vi "Plot strain.vi"() -> ()   [LabVIEW 2015]
uses:
  <vilib>/Utility/file.llb/Read Delimited Spreadsheet (DBL).vi
panel:
  in  "Tab Control":enum32{"Individua strain", "Total strain"}(tab)
  out "XY Graph":cluster{dbl[], "all rows":dbl[]}[](graph)
  out "XY Graph 2":cluster{dbl[], "all rows":dbl[]}[](graph)
  in  "Strain bolt number":i32
  in  "Array":path[](array[path])
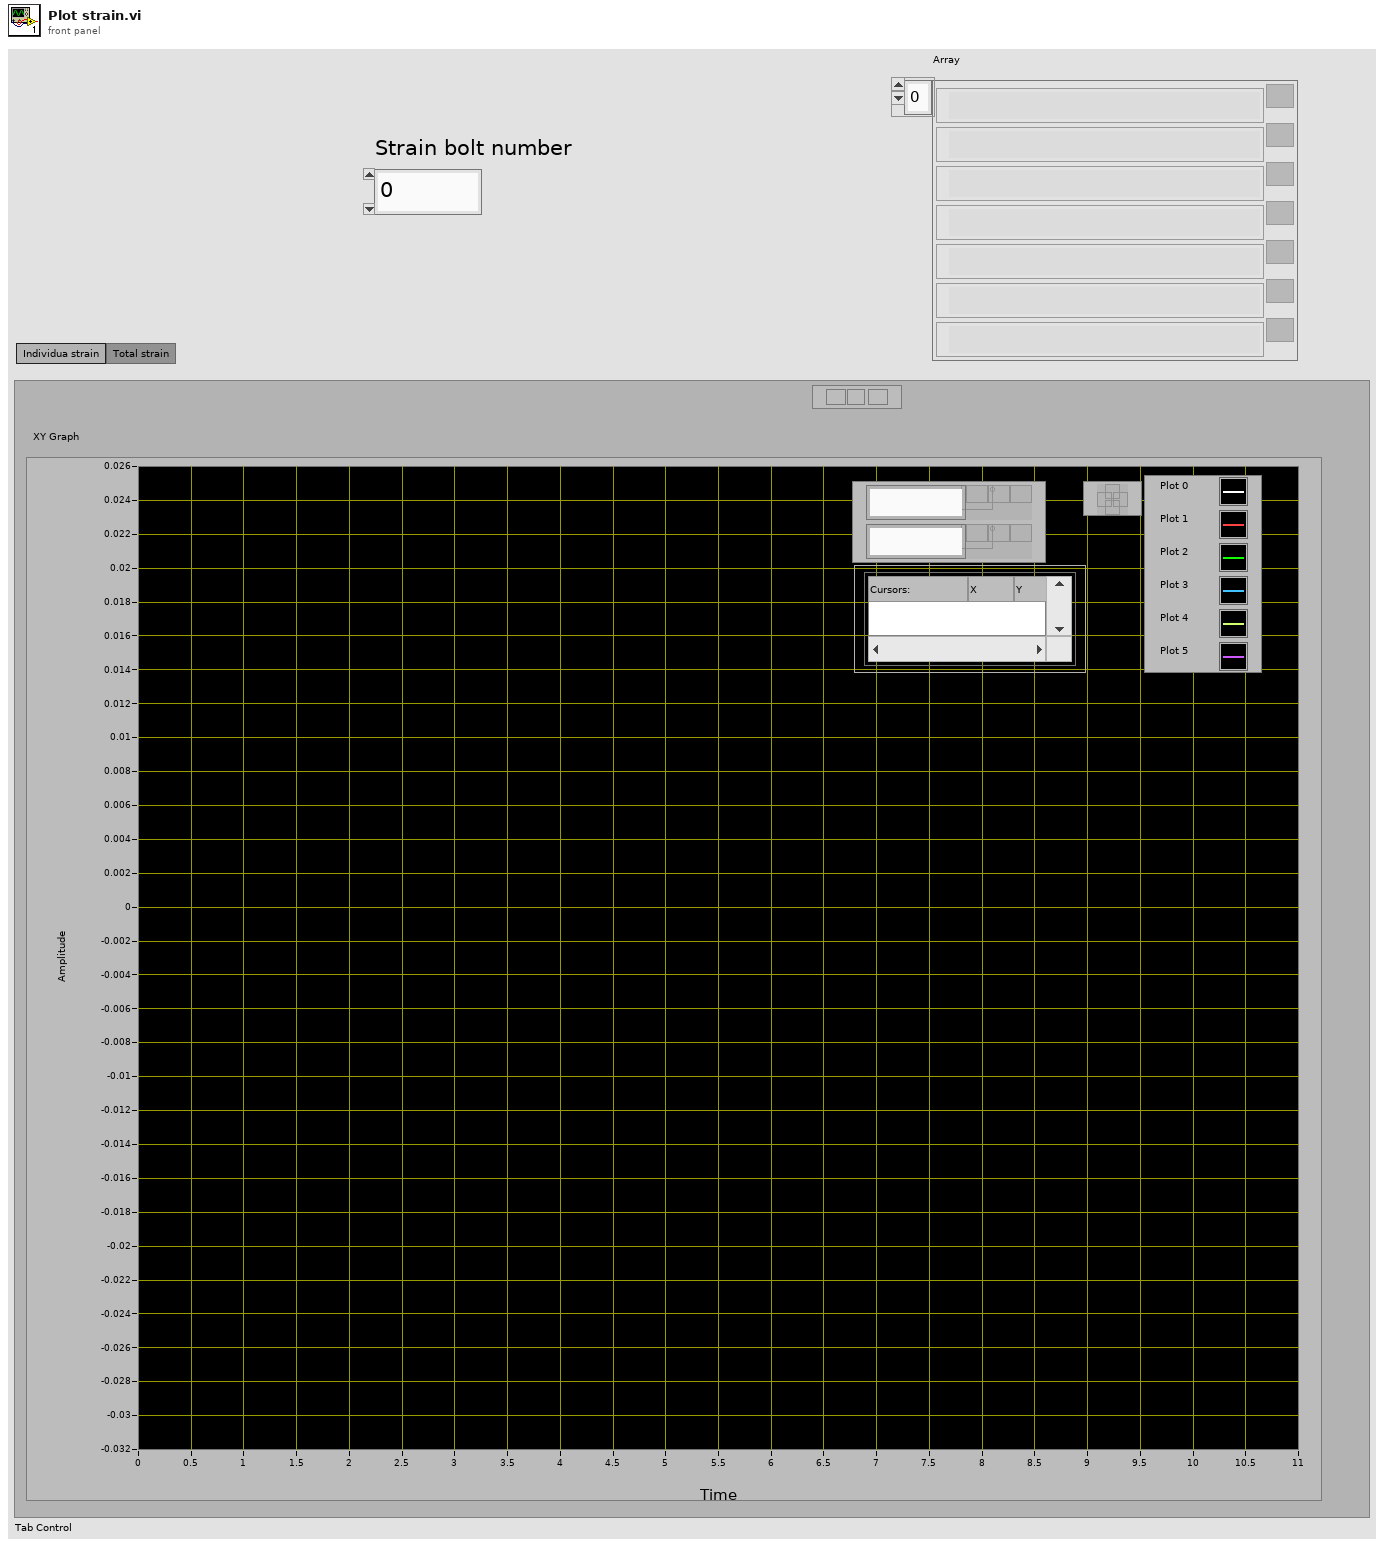
[diagram p1: front panel]
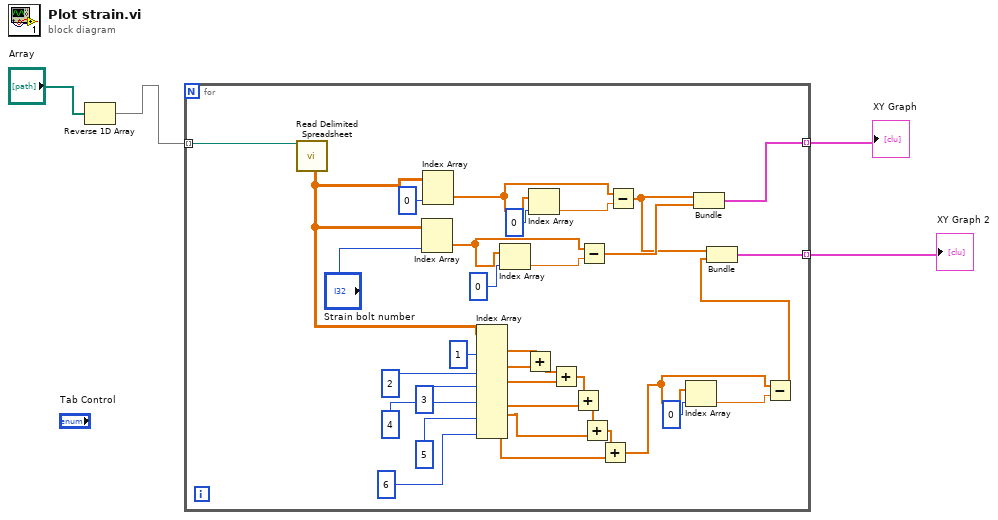
[diagram p0: block diagram]
diagram:
  n1 = Reverse 1D Array(array="Array") -> (reversed array=w2:path[])
  n2 = for {
    tunnel: w2 -> [w31] mode=indexing
    tunnel: [w30] -> w4 mode=indexing
    tunnel: [w26] -> w1 mode=indexing
    n3 = call-poly <vilib>:"Read Delimited Spreadsheet.vi"("file path (dialog if empty)"=w31) -> ("all rows"=w22:dbl[][])  [unwired: 9 in, 5 out]
    n4 = Index Array(array=w22, index (col)="Strain bolt number") -> (element=w32:dbl[])  [unwired: 1 in]
    n5 = Index Array(array=w22, index (col)=0 ("disabled index (col)")) -> (element=w35:dbl[])  [unwired: 1 in]
    n6 = Index Array(array=w22, index (col) #1=1 ("disabled index (col)"), index (col) #2=2 ("index (col)"), index (col) #3=3 ("index (col)"), index (col) #4=4 ("index (col)"), index (col) #5=5 ("index (col)"), index (col) #6=6 ("index (col)")) -> (element #1=w15:dbl[], element #2=w14:dbl[], element #3=w12:dbl[], element #4=w10:dbl[], element #5=w8:dbl[], element #6=w6:dbl[])  [unwired: 6 in]
    n7 = Index Array(array=w32, index=0) -> (element=w33:dbl)
    n8 = Add(x=w15, y=w14) -> (x+y=w13:dbl[])
    n9 = Index Array(array=w35, index=0) -> (element=w36:dbl)
    n10 = Add(x=w13, y=w12) -> (x+y=w11:dbl[])
    n11 = Add(x=w11, y=w10) -> (x+y=w9:dbl[])
    n12 = Subtract(x=w32, y=w33) -> (x-y=w29:dbl[])
    n13 = Add(x=w9, y=w8) -> (x+y=w7:dbl[])
    n14 = Add(x=w7, y=w6) -> (x+y=w5:dbl[])
    n15 = Subtract(x=w35, y=w36) -> (x-y=w27:dbl[])
    n16 = Index Array(array=w5, index=0) -> (element=w24:dbl)
    n17 = Bundle(w27, w29) -> (w30:cluster{dbl[], dbl[]})  [unwired: 1 in]
    n18 = Subtract(x=w5, y=w24) -> (x-y=w23:dbl[])
    n19 = Bundle(w27, w23) -> (w26:cluster{dbl[], dbl[]})  [unwired: 1 in]
  }
  "XY Graph" <- w4
  "XY Graph 2" <- w1
